vi "Image MultiMatch.vi"(7 "Image file paths":path[](array[path]), 11 "Refnum in":T2) -> (1 "num matches":i32[](array[numeric]), 3 "Refnum in 2":T2(plugin-control))   [LabVIEW 2014]
uses:
  <vilib>/vision/Image Controls.llb/IMAQ Image.ctl
  <vilib>/vision/NI_Vision_Development_Module.lvlib
panel:
  in  "Parameters":T1={"Number of Matches Requested"=1, "Minimum Match Score"=800.0, "Angle Ranges"=[]}
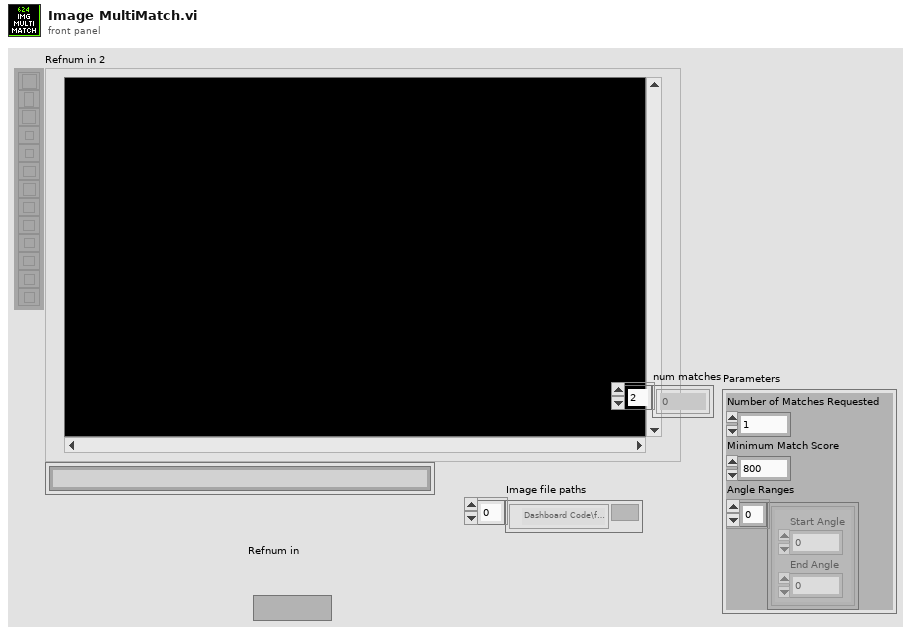
[diagram p1: front panel]
types:
  T1 = cluster{"Number of Matches Requested":i32, "Minimum Match Score":sgl, "Angle Ranges":cluster{"Start Angle":sgl, "End Angle":sgl}[]}
  T2 = typedef "IMAQ Image.ctl" = refnum<image>
  T3 = cluster{"Position":cluster{"x":sgl, "y":sgl}, "Angle":sgl, "Scale":sgl, "Score":sgl, "Bounding Box":cluster{"x":sgl, "y":sgl}[]}
  T4 = typedef "Image Type" = u32
  T5 = cluster{"Position":cluster{"x":sgl, "y":sgl}, "Angle":sgl, "Scale":sgl, "Score":sgl, "Bounding Box":cluster{"x":sgl, "y":sgl}[]}[]
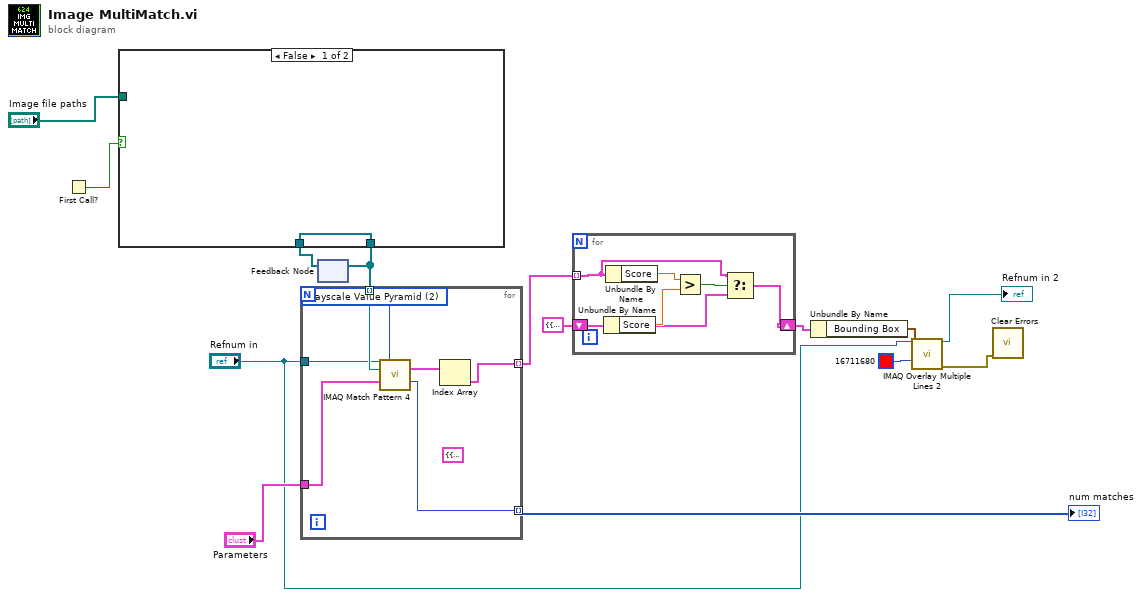
[diagram p0: block diagram]
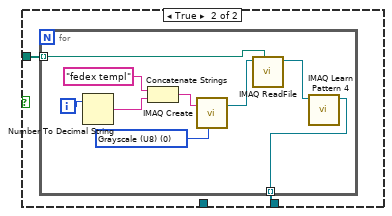
[diagram p2: hidden frame]
diagram:
  n1 = First Call?() -> (First Call?: T/F=w11:bool)
  n2 = feedback #1() -> (w9:T2[])  [unwired: 1 in]
  n3 = case shown="False" w11 {
    tunnel: "Image file paths" -> [_ w17]
    tunnel: [w15 w16] -> w10
    tunnel: w9 -> [w15 _]
    frame False {
    }
    frame True {
      n4 = for {
        tunnel: w17 -> [w20] mode=indexing
        tunnel: [w18] -> w16 mode=indexing
        i -> [w26]
        w23 = T4 0 items=["Grayscale (U8)", "Grayscale (I16)", "Grayscale (SGL)", "Complex (CSG)", "RGB (U32)", "HSL (U32)", "RGB (U64)", "Grayscale (U16)"] ("Image Type")
        n5 = Number To Decimal String(number=w26) -> (decimal integer string=w24:string)  [unwired: 1 in]
        n6 = Concatenate Strings("fedex templ" ("Image Name"), w24) -> (w22:string)
        n7 = call "IMAQ Create"("Image Name"=w22, "Image Type"=w23) -> ("New Image"=w21:T2)  [unwired: 3 in, 1 out]
        n8 = call "IMAQ ReadFile"("File Path"=w20, "Image"=w21) -> ("Image Out"=w19:T2)  [unwired: 5 in, 4 out]
        n9 = call "IMAQ Learn Pattern 4"("Image"=w19) -> ("Template Image Out"=w18:T2)  [unwired: 8 in, 2 out]
      }
    }
  }
  n10 = for {
    tunnel: w10 -> [w33] mode=indexing
    tunnel: "Parameters" -> [w32]
    tunnel: [w31] -> w12 mode=indexing
    tunnel: "Refnum in" -> [w28]
    tunnel: [w27] -> w6 mode=indexing
    (unwired) T3 {"Position"={"x"=0.0, "y"=0.0}, "Angle"=0.0, "Scale"=0.0, "Score"=0.0, "Bounding Box"=[]} ("Match")
    w30 = 2 items=["All", "Low Discrepancy Sampling", "Grayscale Value Pyramid", "Gradients Pyramid"] ("Algorithm")
    n11 = call "IMAQ Match Pattern 4"("Image"=w28, "Algorithm"=w30, "Template Image"=w33, "Parameters"=w32) -> ("Matches (pixel)"=w29:T5, "Number of Matches"=w31:i32)  [unwired: 7 in, 3 out]
    n12 = Index Array(array=w29) -> (element=w27:T3)  [unwired: 1 in]
  }
  "num matches" <- w12
  n13 = feedback-in #1(w10) -> ()
  n14 = for {
    tunnel: w6 -> [w36] mode=indexing
    shift-right: [w34] -> w5
    shift-left: T3 {"Position"={"x"=0.0, "y"=0.0}, "Angle"=0.0, "Scale"=0.0, "Score"=0.0, "Bounding Box"=[]} ("Match") -> [w35]
    n15 = Unbundle By Name(w35) -> ("Score"=w38:sgl)
    n16 = Unbundle By Name(w36) -> ("Score"=w37:sgl)
    n17 = Greater?(x=w37, y=w38) -> (0:w39:bool)
    n18 = Select(t=w36, s=w39, f=w35) -> (s? t:f=w34:T3)
  }
  n19 = Unbundle By Name(w5) -> ("Bounding Box"=w3:cluster{"x":sgl, "y":sgl}[])
  n20 = call "IMAQ Overlay Multiple Lines 2"("Image"="Refnum in", "Line End Points"=w3, "Color"=u32 16711680) -> ("Image Out"=→"Refnum in 2":T2, "error out"=w7:errorcluster)  [unwired: 11 in]
  n21 = call <vilib>:"Clear Errors.vi"("error in (no error)"=w7) -> ()  [unwired: 5 in, 2 out]
